vi "ROS_Topic_Repeat.vi"(3 "error in (no error)":errorcluster, 4 "Msg in":string, 5 "ROS in":T1={"topic port"=0, "Node"="", "topic"="", "type"="", "node port"=0, "error "={"status"=FALSE, "code"=0, "source"=""}, "Direction"=enum."Node", "Update (ms)"=1, "FIFO size"=1}) -> (0 "error out":errorcluster, 2 "ROS out":T1={"topic port"=0, "Node"="", "topic"="", "type"="", "node port"=0, "error "={"status"=FALSE, "code"=0, "source"=""}, "Direction"=enum."Node", "Update (ms)"=1, "FIFO size"=1})   [LabVIEW 2016]
doc: "Prepends the length to Msg in before sending out the data on the specified topic. Use only for publishers and service clients. Messages need to be formatted using Message Building functionality. \n\nSetting Continuous to True will instruct the server to publish the message it received as quickly as possible, updating the message when a new ROS_Topic_Write is called."
uses:
  SubVIs/_ROSControl.ctl
  SubVIs/_ROSDirection.ctl
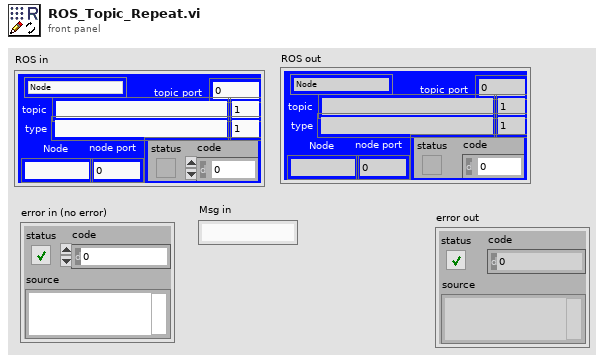
[diagram p1: front panel]
types:
  T1 = typedef "_ROSControl.ctl" = cluster{"topic port":u16, "Node":string, "topic":string, "type":string, "node port":u16, "error ":errorcluster, "Direction":T2, "Update (ms)":u16, "FIFO size":u16}
  T2 = typedef "_ROSDirection.ctl" = enum16{"Node", "Publisher", "Subscriber", "ServiceClient", "ServiceProvider"}
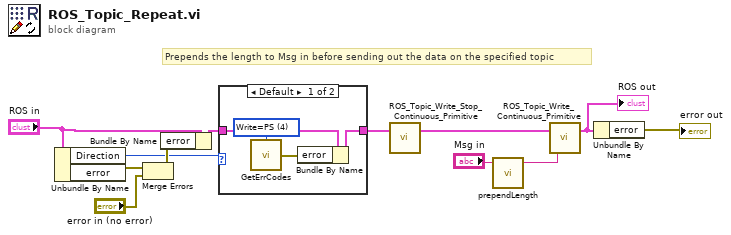
[diagram p0: block diagram]
diagram:
  # "Prepends the length to Msg in before sending out the data on the specified topic"
  n1 = Unbundle By Name("ROS in") -> ("Direction"=w7:T2, "error"=w8:errorcluster)
  n2 = Merge Errors(w8, "error in (no error)") -> (w11:errorcluster)
  n3 = Bundle By Name(cluster="ROS in", "error"=w11) -> (w10:T1)
  n4 = case shown="Default" w7 {
    tunnel: [w16 w17] -> w5
    tunnel: w10 -> [w15 w17]
    frame Default {
      w14 = u16 4 items=["TopicReadTimeout", "Read=SS", "GetQueueErr", "NoMaster", "Write=PS"] ("Error")
      n5 = call "GetErrCodes.vi"("Error"=w14) -> ("Error"=w13:errorcluster)  [unwired: 1 in]
      n6 = Bundle By Name(cluster=w15, "error"=w13) -> (w16:T1)
    }
    frame "Publisher", "ServiceClient" {
    }
  }
  n7 = call "ROS_Topic_Write_Stop_Continuous_Primitive.vi"("ROS in"=w5) -> ("ROS out"=w4:T1)  [unwired: 2 in]
  n8 = call "prependLength.vi"("msg in"="Msg in") -> ("msg out"=w3:string)  [unwired: 4 in]
  n9 = call "ROS_Topic_Write_Continuous_Primitive.vi"("Msg in"=w3, "ROS in"=w4) -> ("ROS out"=w2:T1)  [unwired: 1 in]
  "ROS out" <- w2
  n10 = Unbundle By Name(w2) -> ("error"=→"error out":errorcluster)
